vi "Test RT Acquisition Engine API.vi"() -> ()   [LabVIEW 2021]
doc: "RT Acquisition Engine API Tester."
uses:
  Host-Control's/DIO Data's from RT.ctl
  Host-Control's/AI-Data from RT.ctl
  <vilib>/Utility/error.llb/DialogType.ctl
  RT Acquisition Engine.lvlib
panel:
  out "AI-Info":T1
  out "DO Data's":T2
  in  "Data In":string
  in  "Hardware Info":bool
  in  "Write Data To the RT":bool
  out "last error":errorcluster
  in  "Show Diagram on Init":bool
  in  "Run as Singleton?":bool
  in  "Show Block Diagram":bool
  in  "Refresh Modules":bool
  out "Active Modules":string[](array[string])
  in  "Stop Module":bool
  in  "Select Module":i32(ring)=-1 caption="Select Module\nTo send Request to" items=["All"=-1, "1"=1, "2"=2]
  in  "Run New Module":bool
  in  "Hide Module Panel":bool
  in  "Show Module Panel":bool
  out "Status":string
  # "This VI tests the API for the Module."
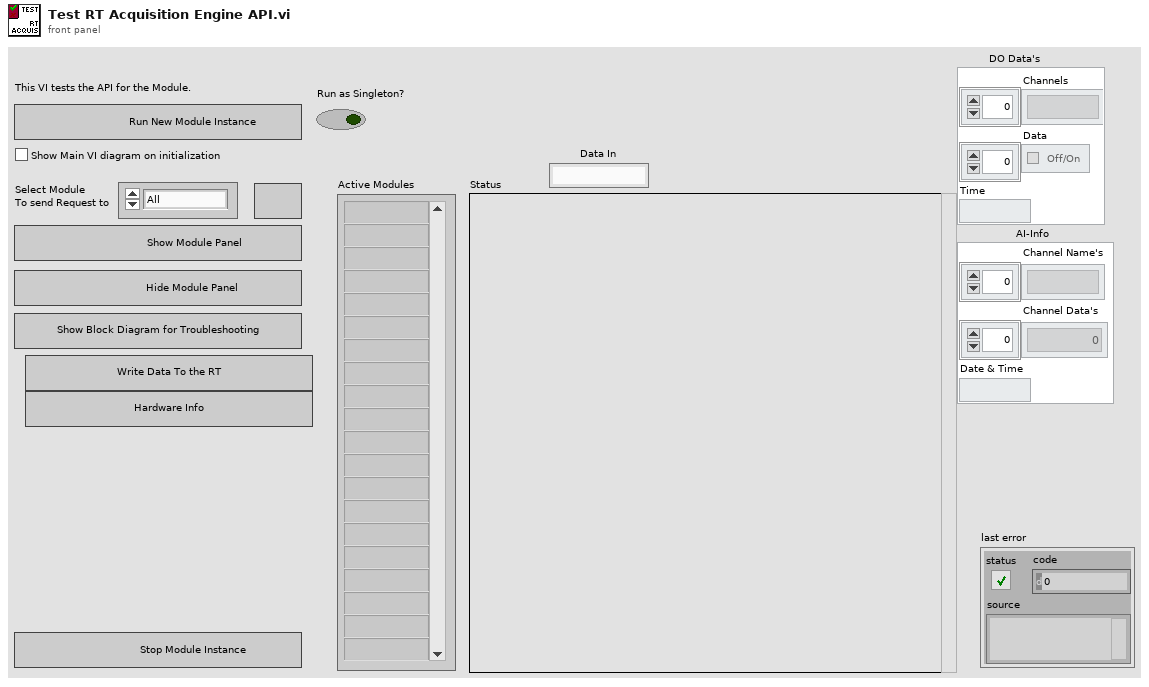
[diagram p1: front panel]
types:
  T1 = typedef "AI-Data from RT.ctl" = cluster{"Channel Name's":string[], "Channel Data's":dbl[], "Date & Time":string}
  T2 = typedef "DIO Data's from RT.ctl" = cluster{"Channels":string[], "Data":bool[], "Time":string}
  T3 = typedef "RT Acquisition Engine.lvlib/Broadcast Events--cluster.ctl" = cluster{"Module Did Init":refnum<user-event>, "Status Updated":refnum<user-event>, "Error Reported":refnum<user-event>, "Module Did Stop":refnum<user-event>, "Update Module Execution Status":refnum<user-event>, "RT Connection Status":refnum<user-event>, "Tx RT Hardware Info":refnum<user-event>, "DO Data's":refnum<user-event>, "AI-Info":refnum<user-event>, "Logging Completed":refnum<user-event>}
  T4 = typedef "DialogType.ctl" = u16
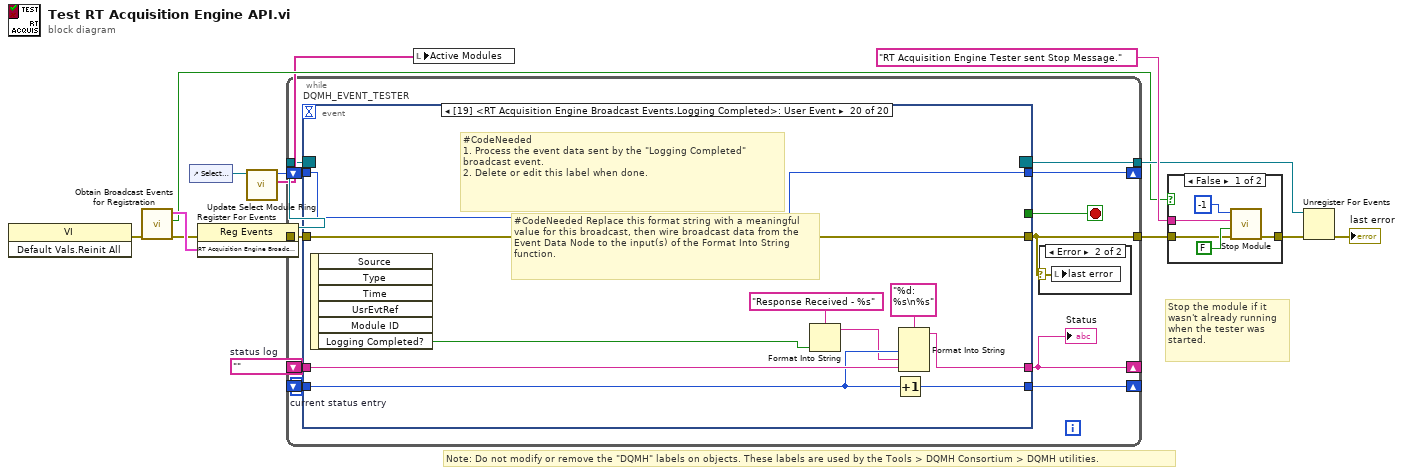
[diagram p0: block diagram]
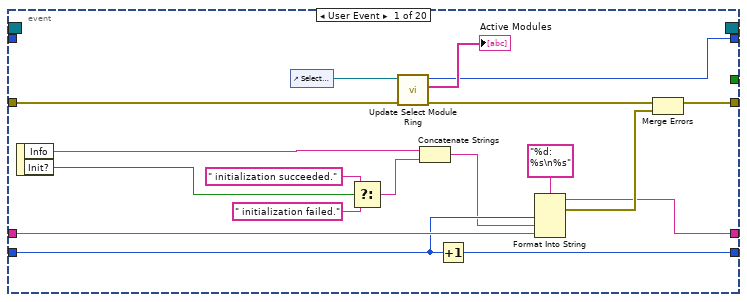
[diagram p4: hidden frame]
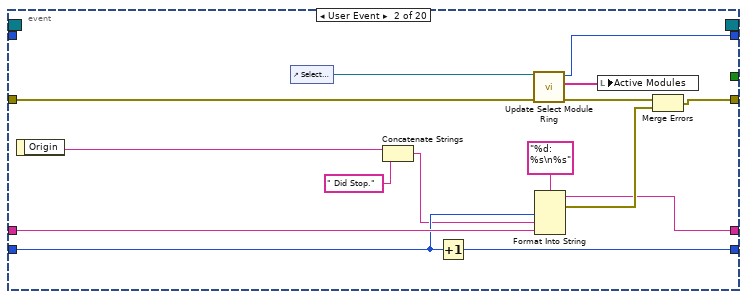
[diagram p5: hidden frame]
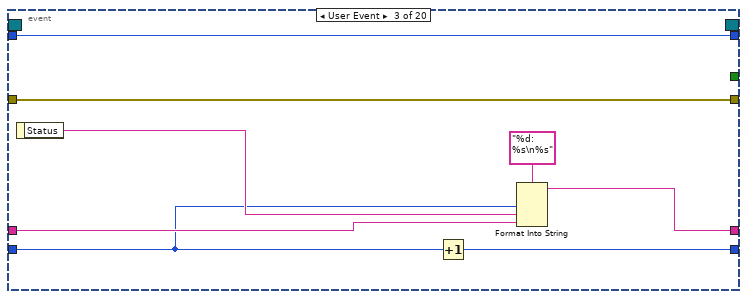
[diagram p6: hidden frame]
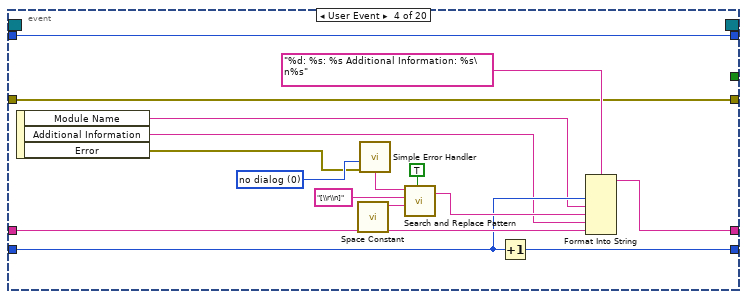
[diagram p7: hidden frame]
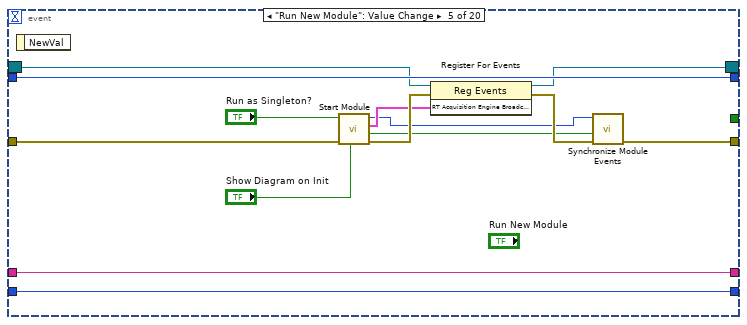
[diagram p8: hidden frame]
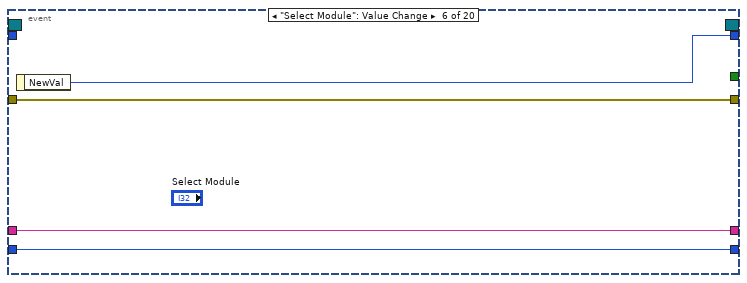
[diagram p9: hidden frame]
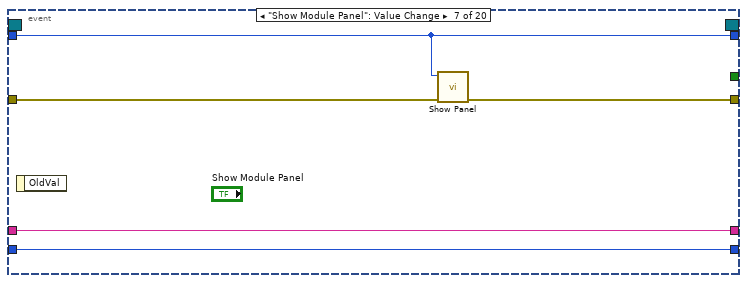
[diagram p10: hidden frame]
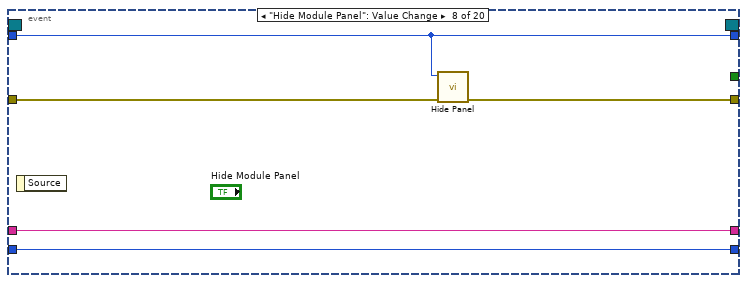
[diagram p11: hidden frame]
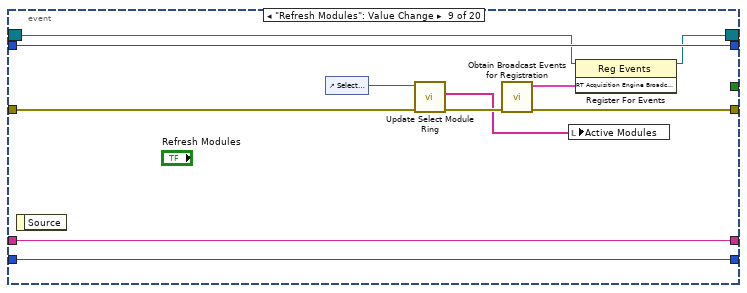
[diagram p12: hidden frame]
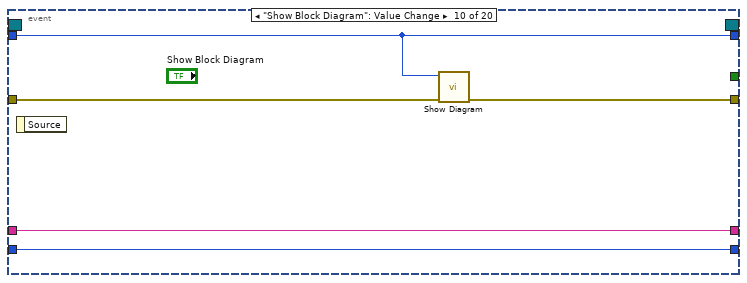
[diagram p13: hidden frame]
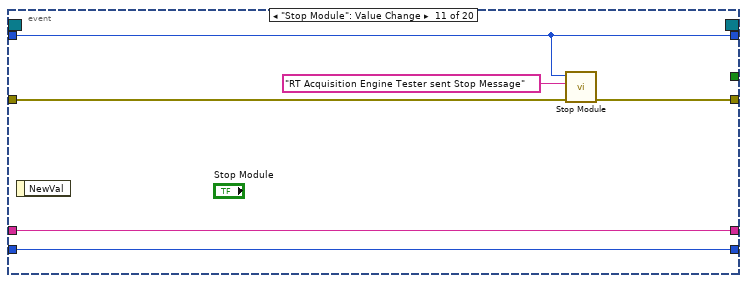
[diagram p14: hidden frame]
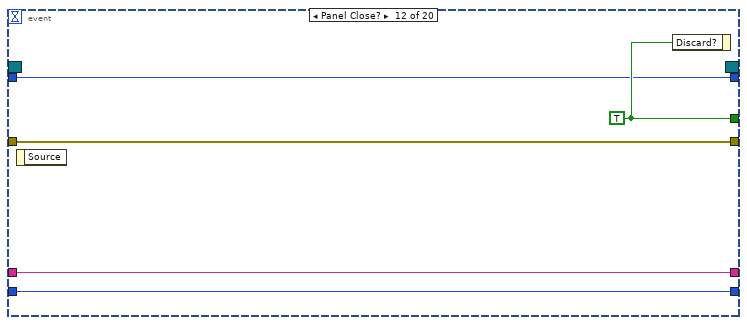
[diagram p15: hidden frame]
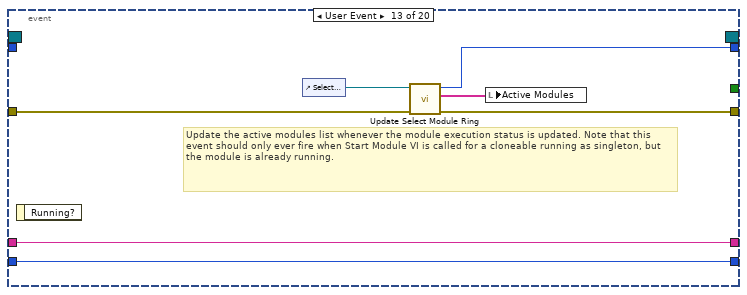
[diagram p16: hidden frame]
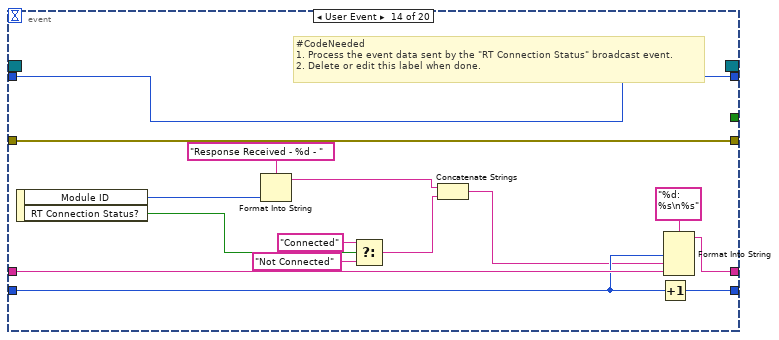
[diagram p17: hidden frame]
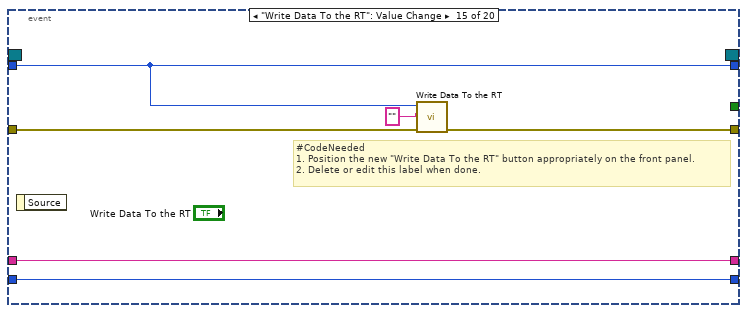
[diagram p18: hidden frame]
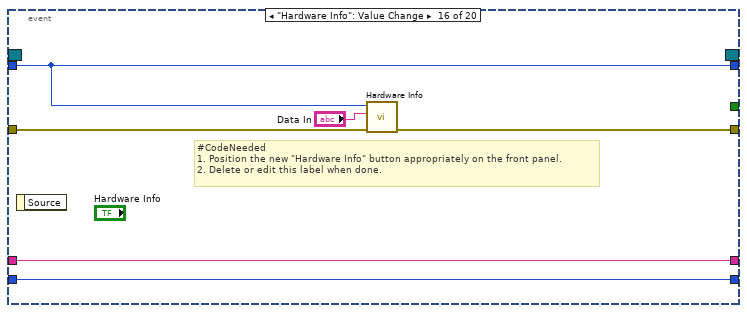
[diagram p19: hidden frame]
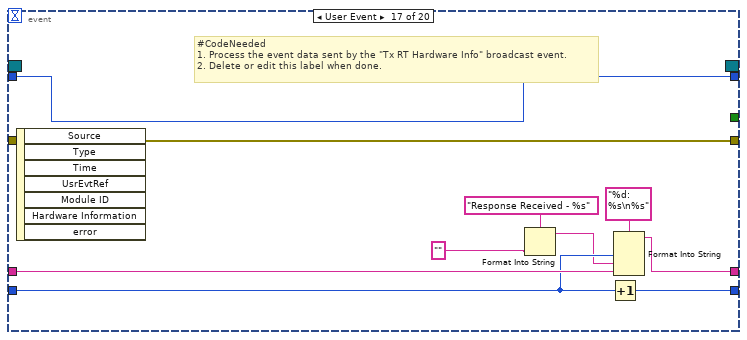
[diagram p20: hidden frame]
diagram:
  w13 = 1  # current status entry
  w14 = ""  # status log
  # "Stop the module if it wasn't already running when the tester was started."
  # "Note: Do not modify or remove the \"DQMH\" labels on objects. These labels are used by the Tools > DQMH Consortium > DQMH utilities."
  n1 = invoke class="VI" method="Default Vals.Reinit All"() -> (error out=w8:errorcluster)  [unwired: 3 in, 2 out]
  n2 = call "Obtain Broadcast Events for Registration.vi"("error in"=w8) -> ("error out"=w7:errorcluster, "Already running?"=w6:bool, "RT Acquisition Engine Broadcast Events"=w12:T3)  [unwired: 8 in]
  n3 = control-ref of="Select Module"() -> (w3:refnum<vi>)
  n4 = register-events(error in=w7, w12) -> (reference out=w16:refnum<event-registration>, error out=w11:errorcluster)  [unwired: 1 in]
  n5 = call "Update Select Module Ring.vi"("Select Module Ring Ref"=w3) -> ("Active Modules (Array)"=w1:string[], "New Module Ring Value"=w2:i32)  [unwired: 8 in, 1 out]
  n6 = while {
    tunnel: w16 -> [w27]
    tunnel: [w18] -> w5
    tunnel: w11 -> [w26]
    shift-right: [w22] -> _
    shift-left: w14 -> [w24]
    shift-right: [w23] -> _
    shift-left: w13 -> [w25]
    shift-right: [w20] -> _
    shift-left: w2 -> [w21]
    tunnel: [w19] -> w9
    stop <- w17 stop-if-true
    n7 = event "DQMH_EVENT_TESTER" shown="[19] <RT Acquisition Engine Broadcast Events.Logging Completed>: User Event" {
      selector: w27 -> [_ _ _ _ w93 _ _ _ w119 _ _ _ _ _ _ _ _ _ _ _]
      dyn-events: [_ _ _ _ w92 _ _ _ w118 _ _ _ _ _ _ _ _ _ _ _] -> w19
      timeout: _ -> [_ _ _ _ _ _ _ _ _ _ _ _ _ _ _ _ _ _ _ _]
      tunnel: [_ _ _ _ _ _ _ _ _ _ _ w140 _ _ _ _ _ _ _ _] -> w17
      tunnel: [w36 w53 w69 w73 w91 w103 w107 w112 w115 w126 w131 w139 w143 w162 w164 w170 w184 w195 w206 w216] -> w18
      tunnel: w26 -> [w38 w55 w69 w73 w94 w103 w108 w113 w120 w129 w132 w139 w144 w162 w168 w174 w184 w195 w206 w216]
      tunnel: w25 -> [w43 w58 w62 w76 w96 w101 w105 w110 w123 w127 w134 w137 w146 w158 w166 w172 w180 w191 w202 w212]
      tunnel: w24 -> [w44 w59 w65 w77 w97 w102 w106 w111 w124 w128 w135 w138 w147 w160 w167 w173 w182 w193 w204 w214]
      tunnel: [w41 w56 w66 w75 w97 w102 w106 w111 w124 w128 w135 w138 w147 w159 w167 w173 w181 w192 w203 w213] -> w22
      tunnel: [w42 w57 w68 w74 w96 w101 w105 w110 w123 w127 w134 w137 w146 w157 w166 w172 w179 w190 w201 w211] -> w23
      tunnel: w21 -> [_ _ w63 w85 w95 _ w104 w109 w122 w125 w133 w136 _ w161 w165 w171 w183 w194 w205 w215]
      tunnel: [w33 w50 w63 w85 w95 w100 w104 w109 w122 w125 w133 w136 w142 w161 w165 w171 w183 w194 w205 w215] -> w20
      event User Event {
        n8 = event-data() -> ("Info"=w40:string, "Init?"=w30:bool)  [unwired: 1 in]
        n9 = control-ref of="Select Module"() -> (w35:refnum<vi>)
        n10 = Select(t=" initialization succeeded.", s=w30, f=" initialization failed.") -> (s? t:f=w29:string)
        n11 = call "Update Select Module Ring.vi"("error in"=w38, "Select Module Ring Ref"=w35) -> ("error out"=w37:errorcluster, "Active Modules (Array)"=→"Active Modules":string[], "New Module Ring Value"=w33:i32)  [unwired: 7 in]
        n12 = Concatenate Strings(w40, w29) -> (w39:string)
        n13 = Increment(x=w43) -> (x+1=w42:i32)
        n14 = Format Into String(format string="%d: %s\n%s", w43, w39, w44) -> (resulting string=w41:string, error out=w46:errorcluster)  [unwired: 2 in]
        n15 = Merge Errors(w37, w46) -> (w36:errorcluster)
      }
      event User Event {
        n16 = event-data() -> ("Origin"=w48:string)  [unwired: 1 in]
        n17 = control-ref of="Select Module"() -> (w52:refnum<vi>)
        n18 = Concatenate Strings(w48, " Did Stop.") -> (w47:string)
        n19 = Increment(x=w58) -> (x+1=w57:i32)
        n20 = call "Update Select Module Ring.vi"("error in"=w55, "Select Module Ring Ref"=w52) -> ("error out"=w54:errorcluster, "Active Modules (Array)"=w51:string[], "New Module Ring Value"=w50:i32)  [unwired: 7 in]
        n21 = Format Into String(format string="%d: %s\n%s", w58, w47, w59) -> (resulting string=w56:string, error out=w61:errorcluster)  [unwired: 2 in]
        n22 = local write "Active Modules"(w51) -> ()
        n23 = Merge Errors(w54, w61) -> (w53:errorcluster)
      }
      event User Event {
        n24 = event-data() -> ("Status"=w64:string)  [unwired: 1 in]
        n25 = Increment(x=w62) -> (x+1=w68:i32)
        n26 = Format Into String(format string="%d: %s\n%s", w62, w64, w65) -> (resulting string=w66:string)  [unwired: 2 in, 1 out]
      }
      event User Event {
        w78 = T4 0 items=["no dialog", "OK message", "continue or stop message", "OK message + warnings", "continue/stop + warnings"] ("type of dialog (OK msg:1)")
        n27 = event-data() -> ("Module Name"=w72:string, "Additional Information"=w71:string, "Error"=w70:errorcluster)  [unwired: 1 in]
        n28 = call <vilib>:"Space Constant.vi"() -> ("String"=w82:string)
        n29 = call <vilib>:"Simple Error Handler.vi"("type of dialog (OK msg:1)"=w78, "error in (no error)"=w70) -> ("message"=w79:string)  [unwired: 3 in, 4 out]
        n30 = call <vilib>:"Search and Replace Pattern.vi"("string"=w79, "regular expression (\"\")"="[\\r\\n]" ("regular expression (\"\")"), "replace string (\"\")"=w82, "replace all? (F)"=TRUE ("replace all CR/LF with spaces")) -> ("result string"=w80:string)  [unwired: 1 in, 1 out]
        n31 = Increment(x=w76) -> (x+1=w74:i32)
        n32 = Format Into String(format string="%d: %s: %s Additional Information: %s\n%s", w76, w72, w80, w71, w77) -> (resulting string=w75:string)  [unwired: 2 in, 1 out]
      }
      event "Run New Module": Value Change {
        n33 = event-data() -> ()  [unwired: 1 in, 1 out]
        n34 = call "Start Module.vi"("Show Main VI Diagram on Init (F)"="Show Diagram on Init", "error in"=w94, "Run as Singleton? (F)"="Run as Singleton?") -> ("error out"=w98:errorcluster, "Wait for Event Sync?"=w90:bool, "RT Acquisition Engine Broadcast Events"=w89:T3, "Module ID"=w86:i32)  [unwired: 5 in]
        n35 = register-events(reference=w93, error in=w98, w89) -> (reference out=w92:refnum<event-registration>, error out=w99:errorcluster)
        n36 = call "Synchronize Module Events.vi"("error in"=w99, "Wait for Event Sync?"=w90, "Module ID in"=w86) -> ("error out"=w91:errorcluster)  [unwired: 7 in, 1 out]
      }
      event "Select Module": Value Change {
        n37 = event-data() -> ("NewVal"=w100:i32)  [unwired: 1 in]
      }
      event "Show Module Panel": Value Change {
        n38 = event-data() -> ()  [unwired: 1 in, 1 out]
        n39 = call "Show Panel.vi"("error in"=w108, "Module ID"=w104) -> ("error out"=w107:errorcluster)  [unwired: 9 in]
      }
      event "Hide Module Panel": Value Change {
        n40 = event-data() -> ()  [unwired: 1 in, 1 out]
        n41 = call "Hide Panel.vi"("error in"=w113, "Module ID"=w109) -> ("error out"=w112:errorcluster)  [unwired: 9 in]
      }
      event "Refresh Modules": Value Change {
        n42 = event-data() -> ()  [unwired: 1 in, 1 out]
        n43 = control-ref of="Select Module"() -> (w121:refnum<vi>)
        n44 = call "Update Select Module Ring.vi"("error in"=w120, "Select Module Ring Ref"=w121) -> ("error out"=w116:errorcluster, "Active Modules (Array)"=w114:string[])  [unwired: 7 in, 1 out]
        n45 = call "Obtain Broadcast Events for Registration.vi"("error in"=w116) -> ("error out"=w115:errorcluster, "RT Acquisition Engine Broadcast Events"=w117:T3)  [unwired: 8 in, 1 out]
        n46 = local write "Active Modules"(w114) -> ()
        n47 = register-events(reference=w119, w117) -> (reference out=w118:refnum<event-registration>)  [unwired: 1 in, 1 out]
      }
      event "Show Block Diagram": Value Change {
        n48 = event-data() -> ()  [unwired: 1 in, 1 out]
        n49 = call "Show Diagram.vi"("error in"=w129, "Module ID"=w125) -> ("error out"=w126:errorcluster)  [unwired: 9 in]
      }
      event "Stop Module": Value Change {
        n50 = event-data() -> ()  [unwired: 1 in, 1 out]
        n51 = call "Stop Module.vi"("error in"=w132, "Origin"="RT Acquisition Engine Tester sent Stop Message", "Module ID"=w133) -> ("error out"=w131:errorcluster)  [unwired: 8 in]
      }
      event Panel Close? {
        w140 = TRUE ("Discard?")
        n52 = event-data() -> ()  [unwired: 1 in, 1 out]
        n53 = event-data("Discard?"=w140) -> ()  [unwired: 1 in, 1 out]
      }
      event User Event {
        # "Update the active modules list whenever the module execution status is updated. Note that this event should only ever fire when Start Module VI is called for a cloneable running as singleton, but the module is already running."
        n54 = event-data() -> ()  [unwired: 1 in, 1 out]
        n55 = control-ref of="Select Module"() -> (w145:refnum<vi>)
        n56 = call "Update Select Module Ring.vi"("error in"=w144, "Select Module Ring Ref"=w145) -> ("error out"=w143:errorcluster, "Active Modules (Array)"=w141:string[], "New Module Ring Value"=w142:i32)  [unwired: 7 in]
        n57 = local write "Active Modules"(w141) -> ()
      }
      event User Event {
        # "#CodeNeeded\n1. Process the event data sent by the \"RT Connection Status\" broadcast event.\n2. Delete or edit this label when done."
        n58 = event-data() -> ("Module ID"=w151:i32, "RT Connection Status?"=w154:bool)  [unwired: 1 in]
        n59 = Format Into String(format string="Response Received - %d - ", w151) -> (resulting string=w150:string)  [unwired: 2 in, 1 out]
        n60 = Select(t="Connected" ("format string"), s=w154, f="Not Connected" ("format string")) -> (s? t:f=w149:string)
        n61 = Concatenate Strings(w150, w149) -> (w148:string)
        n62 = Increment(x=w158) -> (x+1=w157:i32)
        n63 = Format Into String(format string="%d: %s\n%s", w158, w148, w160) -> (resulting string=w159:string)  [unwired: 2 in, 1 out]
      }
      event "Write Data To the RT": Value Change {
        # "#CodeNeeded\n1. Position the new \"Write Data To the RT\" button appropriately on the front panel.\n2. Delete or edit this label when done."
        n64 = event-data() -> ()  [unwired: 1 in, 1 out]
        n65 = call "Write Data To the RT.vi"("error in"=w168, "Data In"="", "Module ID"=w165) -> ("error out"=w164:errorcluster)  [unwired: 8 in]
      }
      event "Hardware Info": Value Change {
        # "#CodeNeeded\n1. Position the new \"Hardware Info\" button appropriately on the front panel.\n2. Delete or edit this label when done."
        n66 = event-data() -> ()  [unwired: 1 in, 1 out]
        n67 = call "Hardware Info.vi"("error in"=w174, "Data In"="Data In", "Module ID"=w171) -> ("error out"=w170:errorcluster)  [unwired: 6 in, 2 out]
      }
      event User Event {
        # "#CodeNeeded\n1. Process the event data sent by the \"Tx RT Hardware Info\" broadcast event.\n2. Delete or edit this label when done."
        n68 = event-data() -> ()  [unwired: 1 in, 7 out]
        n69 = Format Into String(format string="Response Received - %s", "" ("input 1")) -> (resulting string=w176:string)  [unwired: 2 in, 1 out]
        n70 = Increment(x=w180) -> (x+1=w179:i32)
        n71 = Format Into String(format string="%d: %s\n%s", w180, w176, w182) -> (resulting string=w181:string)  [unwired: 2 in, 1 out]
      }
      event User Event {
        # "#CodeNeeded\n1. Process the event data sent by the \"DO Data's\" broadcast event.\n2. Delete or edit this label when done."
        n72 = event-data() -> ("Module ID"=w188:i32, "DO Data's"=→"DO Data's":T2)  [unwired: 1 in]
        n73 = Format Into String(format string="Response Received - %d -", w188) -> (resulting string=w185:string)  [unwired: 2 in, 1 out]
        n74 = Increment(x=w191) -> (x+1=w190:i32)
        n75 = Format Into String(format string="%d: %s\n%s", w191, w185, w193) -> (resulting string=w192:string)  [unwired: 2 in, 1 out]
      }
      event User Event {
        # "#CodeNeeded\n1. Process the event data sent by the \"AI-Info\" broadcast event.\n2. Delete or edit this label when done."
        n76 = event-data() -> ("Module ID"=w197:i32, "AI-Info"=→"AI-Info":T1)  [unwired: 1 in, 4 out]
        n77 = Format Into String(format string="Response Received - %d", w197) -> (resulting string=w198:string)  [unwired: 2 in, 1 out]
        n78 = Increment(x=w202) -> (x+1=w201:i32)
        n79 = Format Into String(format string="%d: %s\n%s", w202, w198, w204) -> (resulting string=w203:string)  [unwired: 2 in, 1 out]
      }
      event User Event {
        # "#CodeNeeded Replace this format string with a meaningful value for this broadcast, then wire broadcast data from the Event Data Node to the input(s) of the Format Into String function."
        # "#CodeNeeded\n1. Process the event data sent by the \"Logging Completed\" broadcast event.\n2. Delete or edit this label when done."
        n80 = event-data() -> ("Logging Completed?"=w207:bool)  [unwired: 1 in, 5 out]
        n81 = Format Into String(format string="Response Received - %s", w207) -> (resulting string=w208:string)  [unwired: 2 in, 1 out]
        n82 = Increment(x=w212) -> (x+1=w211:i32)
        n83 = Format Into String(format string="%d: %s\n%s", w212, w208, w214) -> (resulting string=w213:string)  [unwired: 2 in, 1 out]
      }
    }
    "Status" <- w22
    n84 = case shown="Error" w18 {
      selector: w18 -> [_ w28]
      frame No Error {
      }
      frame Error {
        n85 = local write "last error"(w28) -> ()
      }
    }
  }
  n86 = local write "Active Modules"(w1) -> ()
  n87 = case shown="False" w6 {
    tunnel: [w221 w222] -> w15
    tunnel: "RT Acquisition Engine Tester sent Stop Message." ("Origin") -> [w220 _]
    tunnel: w5 -> [w217 w222]
    frame False {
      n88 = call "Stop Module.vi"("error in"=w217, "Wait for Module to stop? (F)"=FALSE ("Wait for Module to stop?"), "Origin"=w220, "Module ID"=-1 ("Stop all")) -> ("error out"=w221:errorcluster)  [unwired: 7 in]
    }
    frame True {
    }
  }
  n89 = Unregister For Events(event registration refnum=w9, error in=w15) -> (error out=→"last error":errorcluster)
